vi "Main Program.vi"() -> ()   [LabVIEW 2018]
uses:
  State.ctl
  <vilib>/Platform/TimedLoop/XDataNode/timing_clust.ctl
  <vilib>/Platform/TimedLoop/XDataNode/nitl_modes.ctl
  <vilib>/Platform/TimedLoop/XDataNode/wakeup.ctl
  <vilib>/Utility/file.llb/Read Delimited Spreadsheet (DBL).vi
  <vilib>/platform/TimedLoop/XDataNode/XDataNode.xnode
  <vilib>/Platform/TimedLoop/XDataNode/XDNodeRunTimeDep.lvlib
panel:
  out "State":T1
  out "Controller":cluster{"Double":dbl, "Double":dbl}(graph)
  out "Velocity":cluster{"Double":dbl, "Position":dbl}(graph)
  out "Phase":dbl(graph)
  in  "Stop":bool
  in  "file path (dialog if empty)":path
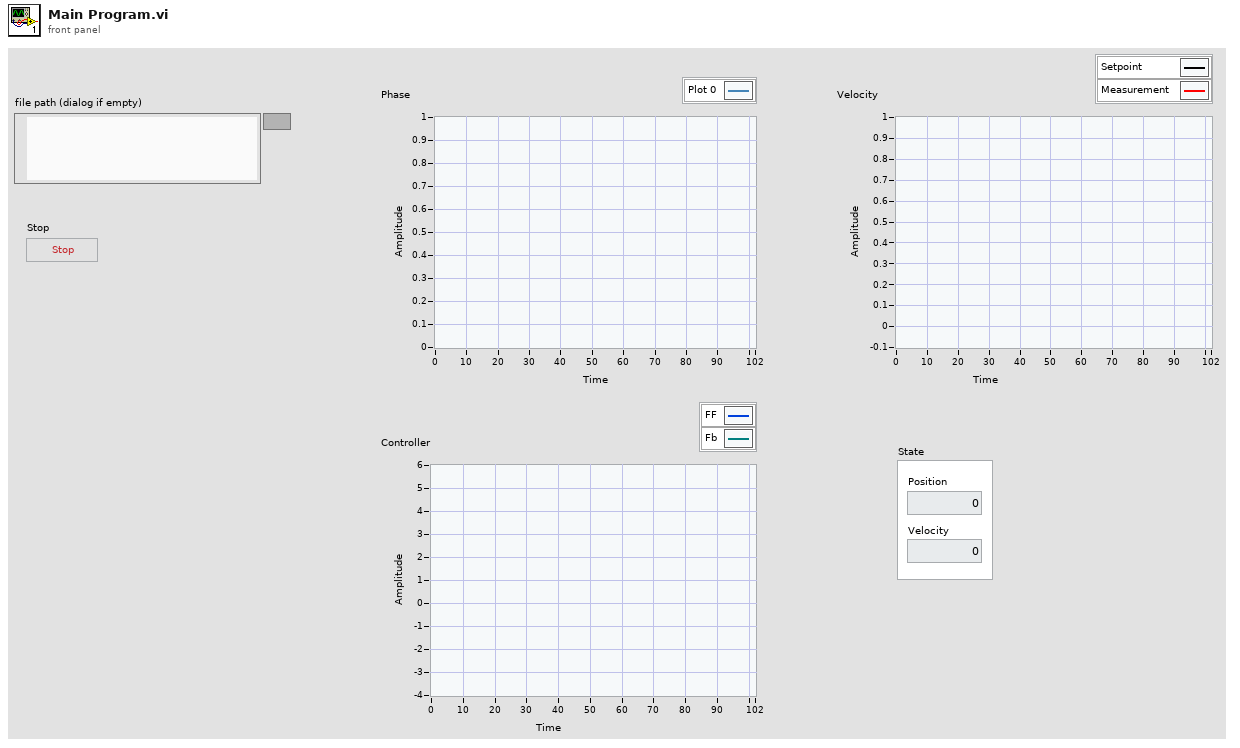
[diagram p1: front panel]
types:
  T1 = typedef "State.ctl" = cluster{"Position":dbl, "Velocity":dbl}
  T2 = typedef "XDNodeRunTimeDep.lvlib/timing_clust.ctl" = cluster{"Expected End [f-1]":u64, "Actual End [f-1]":u64, "Finished Late? [f-1]":bool, "Expected End [i-1]":u64, "Actual End [i-1]":u64, "Finished Late? [i-1]":bool, "Expected Start [i]":u64, "Actual Start [i]":u64, "Expected Start [f]":u64, "Actual Start [f]":u64, "Source Name":string, "Structure Name":string, "Period":i64, "Deadline":i64, "Offset":i64, "Start":i64, "Priority":i32, "Timeout":i32, "Mode":T3, "Wakeup Reason":T4, "Error":errorcluster, "Source Type":string, "Secondary Source Type":string, "Global End Time":u64, "Global Start Time":u64, "Frame Duration":u64, "Iteration Duration":u64, "Assigned CPU":i32, "I/O Scan Engine Mode":u32}
  T3 = typedef "XDNodeRunTimeDep.lvlib/nitl_modes.ctl" = enum32{"No Change", "Process missed periods, maintain original phase", "Discard missed periods, maintain original phase", "Process missed periods, ignore original phase", "Discard missed periods, ignore original phase"}
  T4 = typedef "XDNodeRunTimeDep.lvlib/wakeup.ctl" = enum32{"Normal", "Aborted", "Asynchronous wakeup", "Timing source error", "Timed loop error", "Timeout"}
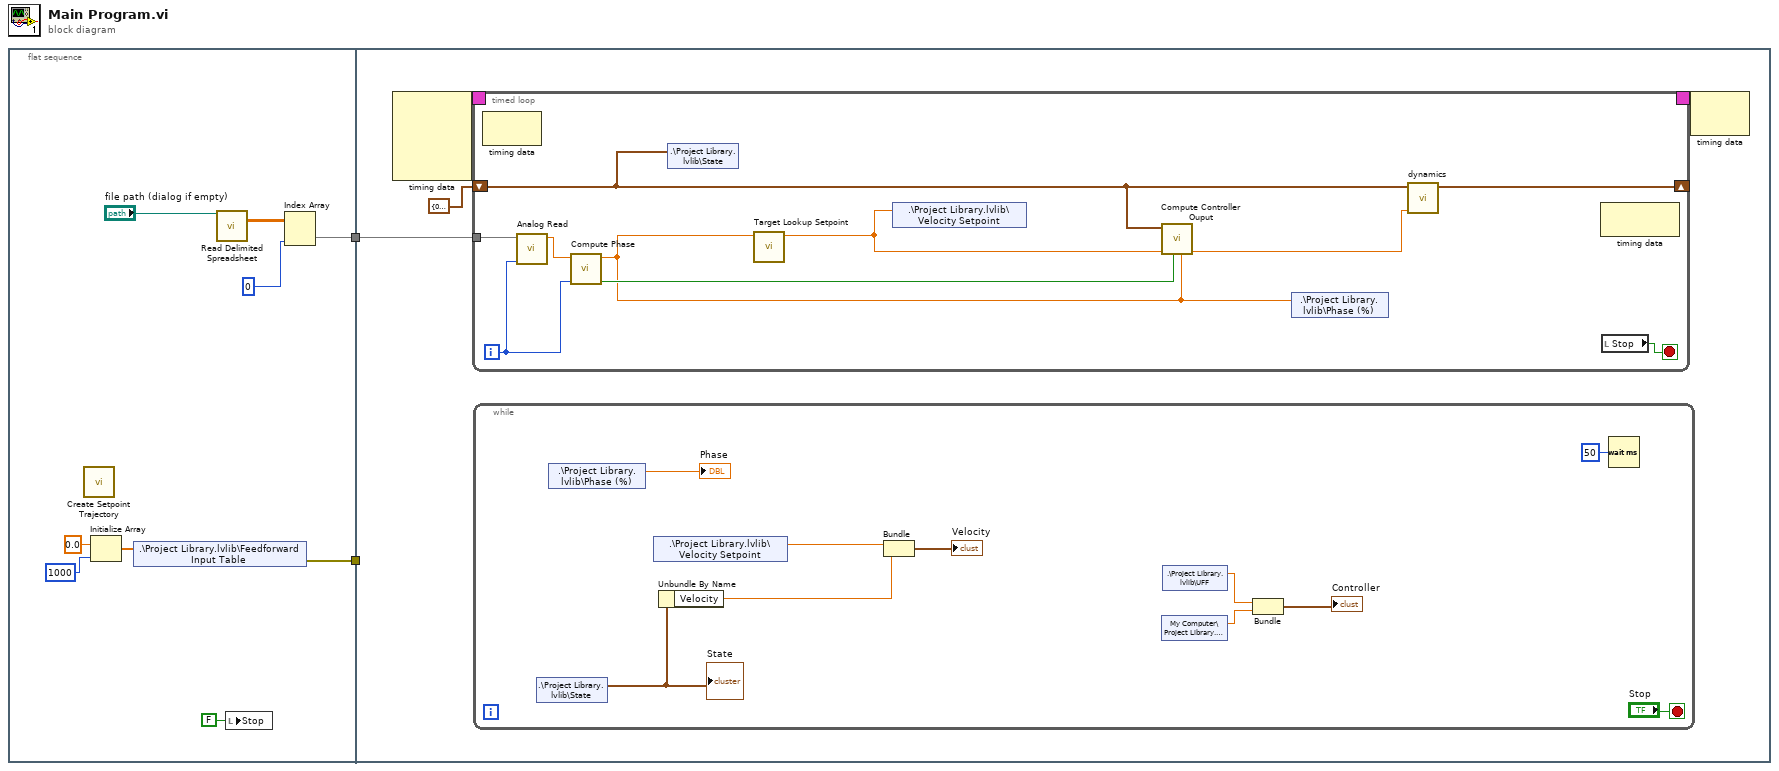
[diagram p0: block diagram]
diagram:
  n1 = flat-sequence {
    tunnel: [w8] -> w2
    tunnel: [w3] -> w1
    tunnel: w2 -> [w13]
    tunnel: w1 -> [_]
    frame #0 {
      n2 = call "Create Setpoint Trajectory.vi"() -> ()  [unwired: 12 in]
      n3 = Initialize Array(0.0 ("element"), 1000 ("dimension size")) -> (w5:dbl[])
      n4 = shared-variable ".\\Project Library.lvlib\\Feedforward Input Table"(w5) -> (error out=w3:errorcluster)  [unwired: 1 in]
      n5 = call-poly <vilib>:"Read Delimited Spreadsheet.vi"("file path (dialog if empty)"="file path (dialog if empty)") -> ("all rows"=w10:dbl[][])  [unwired: 9 in, 5 out]
      n6 = local write "Stop"(FALSE ("Stop")) -> ()
      n7 = Index Array(array=w10, index (col)=0 ("disabled index (col)")) -> (element=w8:dbl[])  [unwired: 1 in]
    }
    frame #1 {
      n8 = node-c288() -> (w15:T2)  [unwired: 4 in]
      n9 = timed-loop {
        timing: w15 -> [_]
        timing-out: [_] -> w14
        tunnel: w13 -> [w34]
        shift-right: [w31] -> _
        shift-left: cluster{"Position":dbl, "Velocity":dbl} {"Position"=0.0, "Velocity"=0.0} ("Future State") -> [w30]
        i -> [w32]
        stop <- w35 stop-if-true
        n10 = node-c288() -> ()  [unwired: 1 in, 1 out]
        n11 = call "Analog Read.vi"("Index"=w32, "Array"=w34) -> ("Force (N)"=w33:dbl)  [unwired: 9 in]
        n12 = call "Compute Phase.vi"("Numeric"=w32, "GRF"=w33) -> ("HS"=w29:bool, "Phase"=w26:dbl)  [unwired: 8 in]
        n13 = shared-variable ".\\Project Library.lvlib\\State"(w30) -> ()  [unwired: 1 in, 1 out]
        n14 = call "Target Lookup Setpoint.vi"("Phase"=w26) -> ("Setpoint"=w28:dbl)  [unwired: 10 in]
        n15 = shared-variable ".\\Project Library.lvlib\\Velocity Setpoint"(w28) -> ()  [unwired: 1 in, 1 out]
        n16 = call "Compute Controller Ouput.vi"("Phase"=w26, "HS"=w29, "Setpoint"=w28, "State"=w30) -> ("Full Output"=w27:dbl)  [unwired: 7 in]
        n17 = shared-variable ".\\Project Library.lvlib\\Phase (%)"(w26) -> ()  [unwired: 1 in, 1 out]
        n18 = call "dynamics.vi"("Control Input"=w27, "State"=w30) -> ("Future State"=w31:cluster{"Position":dbl, "Velocity":dbl})  [unwired: 9 in]
        n19 = node-c288() -> ()  [unwired: 1 in, 1 out]
        n20 = local read "Stop"() -> (w35:bool)
      }
      n21 = while {
        stop <- "Stop" stop-if-true
        n22 = shared-variable ".\\Project Library.lvlib\\State"() -> (w22:T1)  [unwired: 1 in, 1 out]
        "State" <- w22
        n23 = shared-variable ".\\Project Library.lvlib\\Phase (%)"() -> (→"Phase":dbl)  [unwired: 1 in, 1 out]
        n24 = shared-variable ".\\Project Library.lvlib\\Velocity Setpoint"() -> (w21:dbl)  [unwired: 1 in, 1 out]
        n25 = Unbundle By Name(w22) -> ("Velocity"=w20:dbl)
        n26 = Bundle("Double"=w21, "Velocity"=w20) -> (→"Velocity":cluster{"Double":dbl, "Velocity":dbl})  [unwired: 1 in]
        n27 = shared-variable "My Computer\\Project Library.lvlib\\UFB"() -> (w17:dbl)  [unwired: 1 in, 1 out]
        n28 = shared-variable ".\\Project Library.lvlib\\UFF"() -> (w18:dbl)  [unwired: 1 in, 1 out]
        n29 = Bundle("Double"=w18, "Double"=w17) -> (→"Controller":cluster{"Double":dbl, "Double":dbl})  [unwired: 1 in]
        n30 = Wait (ms)(milliseconds to wait=u32 50) -> ()  [unwired: 1 out]
      }
      n31 = node-c288(w14) -> ()  [unwired: 1 out]
    }
  }
